vi "Fgen Basic Arb Waveform.vi"() -> ()   [LabVIEW 2021]
doc: "This example shows how to use Arbitrary Waveform mode. This is a basic example that shows the smallest amount of code necessary to generate an arbitrary waveform."
uses:
  <instrlib>/niFgen/niFgen.llb/niFgen Output Mode.ctl
  <instrlib>/niFgen/niFgen.llb/niFgen Create Waveform (I16).vi
panel:
  in  "Waveform Information":T1={"Waveform Type"=0, "Amplitude"=1.0, "# of points"=256} {"Amplitude" min=0.0 max=1.0 format="%.2f"; "Waveform Type" items=["Sine", "Cosine", "Triangle", "Square", "Sawtooth", "Increasing Ramp", "Decreasing Ramp", "DC Value"]}
  in  "DC Offset":dbl(knob) scale=-0.5..0.5 scale format="%#.1f"
  in  "Gain":dbl(knob)=1.0 min=0.0 max=5.0 scale=0.0..5.0 scale format="%#.1f"
  in  "FGEN Resource Name":refnum<k15>
  in  "Stop":bool
  # "Overview: Demonstrates how to configure an NI Arbitrary Waveform Generator to generate a basic arbitrary waveform with Arbitrary Waveform Mode.\nSoftware Requirements: NI-FGEN\nHardware Requirements: PXI-5411, PCI-5411, AT-5411, PXI-5412, PCI-5412, PXIe-5413, PXI-5421, PCI-5421, PXI-5422, PXIe-5423, PXI-5431, PCI-5431, PXIe-5433, PXI-5441, NI PXIe-5442, NI PXIe-5450, or NI PXIe-5451 \nInstructions:\n1. Select the FGEN Resource Name as configured in the Measurement & Automation Explorer.\n2. Specify the waveforms that will be generated in the Waveform Information.\n3. Specify the Gain that will be used.\n4. Select the DC Offset that will be used.\n5. Run the VI.\n6. Click Stop to stop the VI."
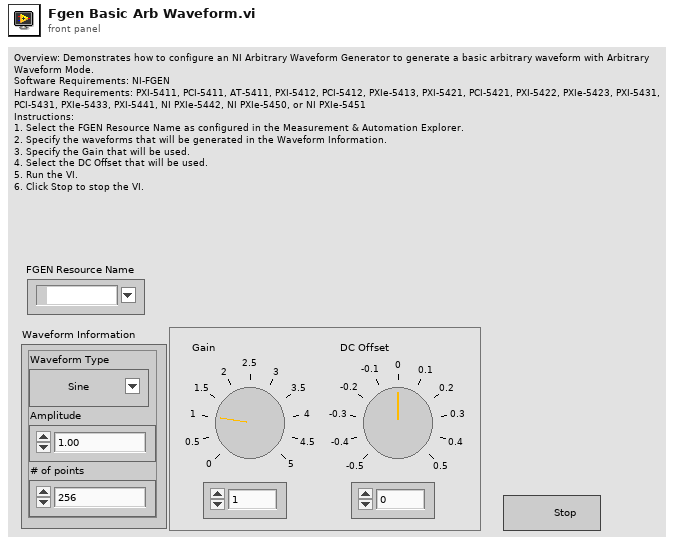
[diagram p1: front panel]
types:
  T1 = cluster{"Waveform Type":u16, "Amplitude":dbl, "# of points":u32}
  T2 = typedef "niFgen Output Mode.ctl" = u32
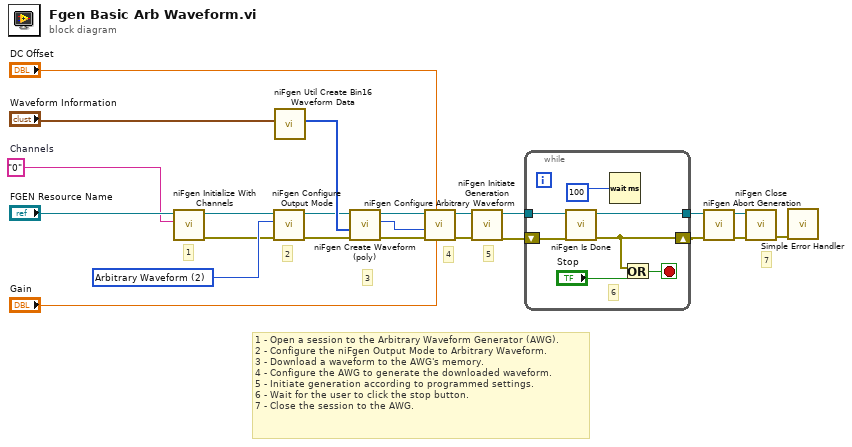
[diagram p0: block diagram]
diagram:
  w1 = "0"  # Channels
  w18 = T2 2 items=["Standard Function", "Frequency List", "Arbitrary Waveform", "Arbitrary Sequence", "Script"] ("output mode")
  # "5"
  # "4"
  # "3"
  # "2"
  # "1"
  # "7"
  # "1 - Open a session to the Arbitrary Waveform Generator (AWG).\n2 - Configure the niFgen Output Mode to Arbitrary Waveform.\n3 - Download a waveform to the AWG's memory.\n4 - Configure the AWG to generate the downloaded waveform.\n5 - Initiate generation according to programmed settings.\n6 - Wait for the user to click the stop button.\n7 - Close the session to the AWG."
  n1 = call <instrlib>:"niFgen Initialize With Channels.vi"("Channel Name"=w1, "Resource Name"="FGEN Resource Name") -> ("error out"=w4:errorcluster, "Instrument Handle Out"=w3:refnum<k15>)  [unwired: 8 in]
  n2 = call <instrlib>:"niFgen Configure Output Mode.vi"("error in (no error)"=w4, "Output Mode (default: 0=Standard Function)"=w18, "Instrument Handle"=w3) -> ("error out"=w19:errorcluster, "Instrument Handle Out"=w20:refnum<k15>)  [unwired: 6 in]
  n3 = call <instrlib>:"niFgen Util Create Bin16 Waveform Data.vi"("Waveform"="Waveform Information") -> ("Waveform Data"=w21:i16[])  [unwired: 10 in]
  n4 = call-poly <instrlib>:"niFgen Create Waveform (poly).vi"("error in (no error)"=w19, "Waveform Data Array"=w21, "Instrument Handle"=w20) -> ("error out"=w14:errorcluster, "Waveform Handle"=w13:i32, "Instrument Handle Out"=w15:refnum<k15>)  [unwired: 6 in]
  n5 = call <instrlib>:"niFgen Configure Arbitrary Waveform.vi"("Gain"="Gain", "Offset"="DC Offset", "error in (no error)"=w14, "Waveform Handle"=w13, "Instrument Handle"=w15) -> ("error out"=w17:errorcluster, "Instrument Handle Out"=w16:refnum<k15>)  [unwired: 5 in]
  n6 = call <instrlib>:"niFgen Initiate Generation.vi"("error in (no error)"=w17, "Instrument Handle"=w16) -> ("error out"=w22:errorcluster, "Instrument Handle Out"=w23:refnum<k15>)  [unwired: 8 in]
  n7 = while {
    tunnel: w23 -> [w27]
    tunnel: [w26] -> w7
    shift-right: [w25] -> w8
    shift-left: w22 -> [w24]
    stop <- w29 stop-if-true
    # "6"
    n8 = call <instrlib>:"niFgen Is Done.vi"("error in (no error)"=w24, "Instrument Handle"=w27) -> ("error out"=w25:errorcluster, "Instrument Handle Out"=w26:refnum<k15>)  [unwired: 7 in, 1 out]
    n9 = Wait (ms)(milliseconds to wait=u32 100 ("millisecond multiple")) -> ()  [unwired: 1 out]
    n10 = Or(x=w25, y="Stop") -> (x .or. y?=w29:bool)
  }
  n11 = call <instrlib>:"niFgen Abort Generation.vi"("error in (no error)"=w8, "Instrument Handle"=w7) -> ("error out"=w5:errorcluster, "Instrument Handle Out"=w6:refnum<k15>)  [unwired: 8 in]
  n12 = call <instrlib>:"niFgen Close.vi"("error in (no error)"=w5, "Instrument Handle"=w6) -> ("error out"=w12:errorcluster)  [unwired: 9 in]
  n13 = call <vilib>:"Simple Error Handler.vi"("error in (no error)"=w12) -> ()  [unwired: 4 in, 5 out]
